vi "Get Main Frame Limits.vi"(6 "Width":u32, 11 "Game Board in":refnum<class "Game Board.lvclass">) -> (2 "rect out":T1(array[cluster]))   [LabVIEW 2021, in "Game Board.lvclass"]
doc: "MIT Licence\nCopyright (c) 2024 David Grollier"
uses:
  Game Board.lvclass
  Game Board.lvclass/Game Board.ctl
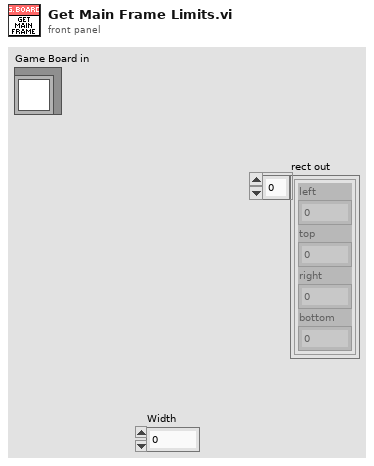
[diagram p1: front panel]
types:
  T1 = cluster{"left":i16, "top":i16, "right":i16, "bottom":i16}[]
  T2 = cluster{"left":i32, "top":i16, "right":i32, "bottom":i32}
  T3 = cluster{"left":i32, "top":i16, "right":i32, "bottom":i32}[]
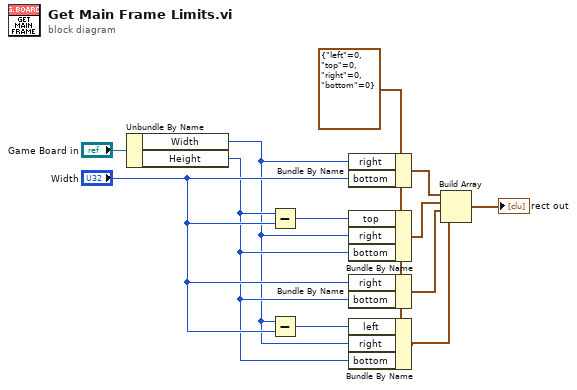
[diagram p0: block diagram]
diagram:
  w12 = T2 {"left"=0, "top"=0, "right"=0, "bottom"=0} ("rect in")
  n1 = Unbundle By Name("Game Board in") -> ("Width"=w1:u32, "Height"=w2:u32)
  n2 = Subtract(x=w2, y="Width") -> (x-y=w6:u32)
  n3 = Subtract(x=w1, y="Width") -> (x-y=w4:u32)
  n4 = Bundle By Name(cluster=w12, "right"=w1, "bottom"="Width") -> (w11:T2)
  n5 = Bundle By Name(cluster=w12, "top"=w6, "right"=w1, "bottom"=w2) -> (w10:T2)
  n6 = Bundle By Name(cluster=w12, "right"="Width", "bottom"=w2) -> (w9:T2)
  n7 = Bundle By Name(cluster=w12, "left"=w4, "right"=w1, "bottom"=w2) -> (w8:T2)
  n8 = Build Array(w11, w10, w9, w8) -> (→"rect out":T3)
